vi "lab10.vi"() -> ()   [LabVIEW 2017]
uses:
  <vilib>/addons/Control Design/_Model Construction/Model Creation.llb/Model Creation SubVI/cd_Create Transfer Function Model.vi
  <vilib>/addons/Control Design/_Frequency Response Analysis/Frequency Response.llb/Frequency Response subVI/cd_Gain and Phase Margin (Transfer Function).vi
  <vilib>/addons/Control Design/_Dynamic Analysis/Dynamic Analysis.llb/Dynamic Analysis subVI/cd_Stability (Transfer Function).vi
  <vilib>/addons/Control Design/_Dynamic Analysis/Dynamic Analysis.llb/Dynamic Analysis subVI/cd_Pole-Zero Map (Transfer Function).vi
  <vilib>/addons/Control Design/_Utility/Model Viewer.llb/Model Viewer SubVI/cd_Draw Transfer Function Equation (TF).vi
  <vilib>/addons/Control Design/_Frequency Response Analysis/Frequency Response.llb/Frequency Response subVI/cd_Bode (Transfer Function).vi
  <vilib>/addons/Control Design/_Frequency Response Analysis/Frequency Response.llb/Frequency Response subVI/cd_Bandwidth (Transfer Function).vi
  <vilib>/addons/Control Design/_Model Construction/NI_LinSys_Model Creation.lvlib
  <vilib>/addons/Control Design/_Frequency Response Analysis/NI_CD_Frequency Response.lvlib
  <vilib>/addons/Control Design/_Utility/NI_CD_Model Viewer.lvlib
  <vilib>/addons/Control Design/_Dynamic Analysis/NI_CD_Dynamic Analysis.lvlib
panel:
  in  "stop":bool
  out "DC Phase Plot":cluster{"W":dbl[], "Phase":dbl[]}[](graph)
  out "DC Gain Magnitude graph":cluster{"W":dbl[], "Magnitude":dbl[]}[](graph)
  out "Stability":T1(ring)=enum."undetermined"
  out "Pole-Zero Map":cluster{dbl[], dbl[]}[](graph)
  out "Equation":picture
  out "Bode Phase":cluster{"W":dbl[], "Magnitude":dbl[]}[](graph)
  out "Bode Magnitude":cluster{"W":dbl[], "Magnitude":dbl[]}[](graph)
  out "Bandwidth":dbl=nan format="%.4f"
  in  "Denominator":dbl[](array[numeric]) format="%#.5g"
  in  "Numerator":dbl[](array[numeric]) format="%#.5g"
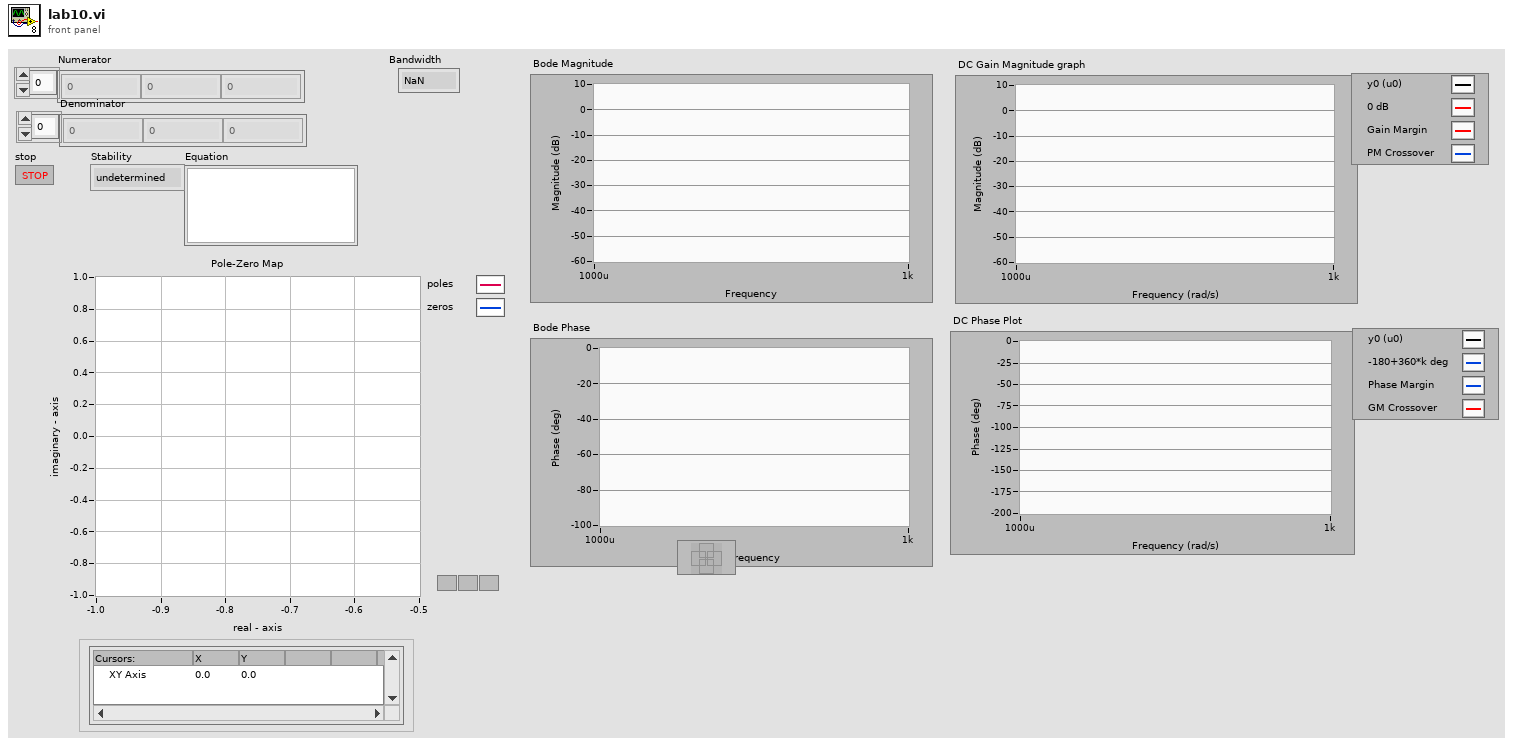
[diagram p1: front panel]
types:
  T1 = enum16{"stable", "marginally stable", "unstable", "undetermined"}
  T2 = typedef "NI_LinSys_Model Typedefs.lvlib/CD Transfer Function Model (MIMO).ctl" = cluster{"properties":T3, "transfer function(s)":T4[][]}
  T3 = typedef "NI_LinSys_Model Typedefs.lvlib/CD General Elements.ctl" = cluster{"Model name":string, "Input names":string[], "Output names":string[], "Input Delays":dbl[], "Output Delays":dbl[], "Sampling Time":dbl, "Notes":string}
  T4 = typedef "NI_LinSys_Model Typedefs.lvlib/CD Transfer Function Model (SISO).ctl" = cluster{"Numerator":dbl[], "Denominator":dbl[], "delay":dbl}
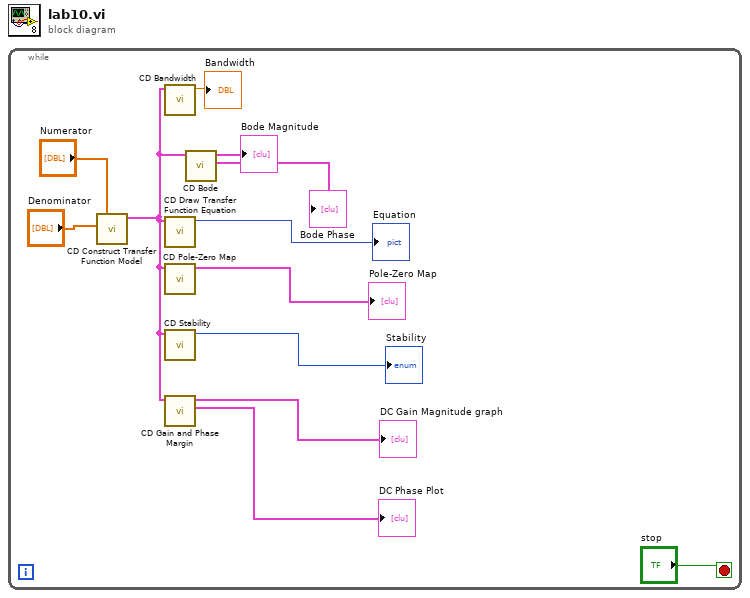
[diagram p0: block diagram]
diagram:
  n1 = while {
    stop <- "stop" stop-if-true
    n2 = call-poly <vilib>:"CD Construct Transfer Function Model.vi"("Denominator"="Denominator", "Numerator"="Numerator") -> ("Transfer Function Model"=w12:T2)  [unwired: 8 in, 1 out]
    n3 = call-poly <vilib>:"CD Bandwidth.vi"("Transfer Function Model"=w12) -> ("Bandwidth"=→"Bandwidth":dbl)  [unwired: 9 in, 1 out]
    n4 = call-poly <vilib>:"CD Draw Transfer Function Equation.vi"("Transfer Function Model"=w12) -> ("Equation"=→"Equation":picture)  [unwired: 8 in, 2 out]
    n5 = call-poly <vilib>:"CD Pole-Zero Map.vi"("Transfer Function Model"=w12) -> ("Pole-Zero Map"=→"Pole-Zero Map":cluster{dbl[], dbl[]}[])  [unwired: 7 in, 3 out]
    n6 = call-poly <vilib>:"CD Stability.vi"("Transfer Function Model"=w12) -> ("Stability"=→"Stability":T1)  [unwired: 8 in, 2 out]
    n7 = call-poly <vilib>:"CD Gain and Phase Margin.vi"("Transfer Function Model"=w12) -> ("Phase Plot"=→"DC Phase Plot":cluster{"W":dbl[], "Phase":dbl[]}[], "Magnitude Plot"=→"DC Gain Magnitude graph":cluster{"W":dbl[], "Magnitude":dbl[]}[])  [unwired: 6 in, 3 out]
    n8 = call-poly <vilib>:"CD Bode.vi"("Transfer Function Model"=w12) -> ("Bode Phase"=→"Bode Phase":cluster{"W":dbl[], "Magnitude":dbl[]}[], "Bode Magnitude"=→"Bode Magnitude":cluster{"W":dbl[], "Magnitude":dbl[]}[])  [unwired: 6 in, 3 out]
  }
